vi "Build Get Type.vi"(8 "error in (no error)":errorcluster, 10 "Get Type VI":refnum<vi>, 11 "CS++Actor in":refnum<class "CS++Actor.lvclass">) -> (0 "error out":errorcluster, 3 "CS++Actor out":refnum<class "CS++Actor.lvclass">)   [LabVIEW 2014, in "CS++Actor.lvlib" / "CS++Actor.lvclass"]
uses:
  CS++Actor.lvclass
  CS++Actor.lvclass/CS++Actor.ctl
  <vilib>/Utility/traverseref.llb/TRef TravTarget.ctl
  <vilib>/Utility/traverseref.llb/VI Scripting - Traverse.lvlib
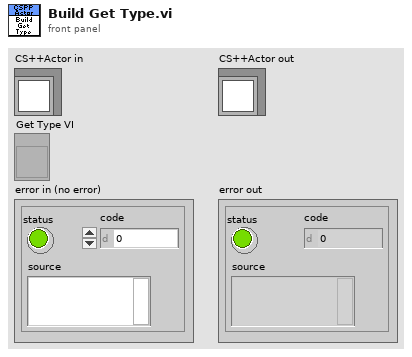
[diagram p1: front panel]
types:
  T1 = enum16{"Replace Class Controls/Indicator", "Connect Unbundler & Bundler"}
  T2 = enum16{"Invalid Wire Rule", "Required", "Recommended", "Optional", "Dynamic Dispatch"}
  T3 = typedef "TRef TravTarget.ctl" = enum16{"FP", "BD", "Other"}
  T4 = typedef "LVRectTypeDef.ctl" = cluster{"Left":i16, "Top":i16, "Right":i16, "Bottom":i16}
  T5 = enum16{"Invalid Wire Rule", "Required", "Recommended", "Optional", "Dynamic Dispatch"}[]
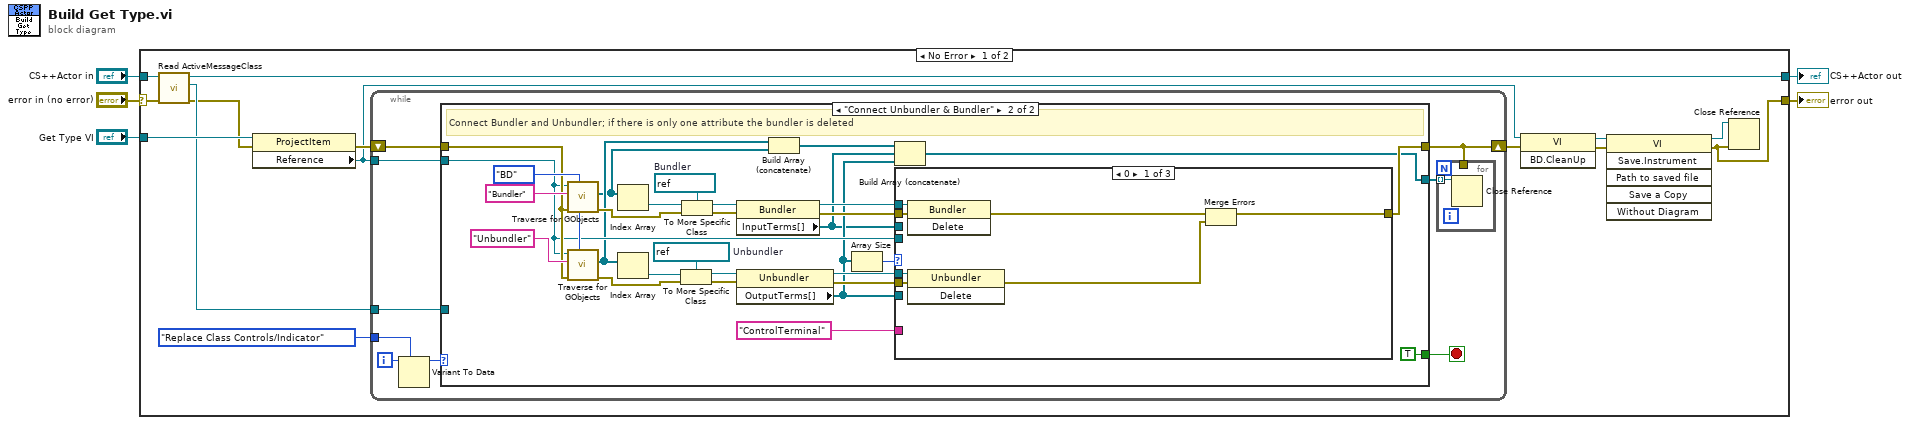
[diagram p0: block diagram]
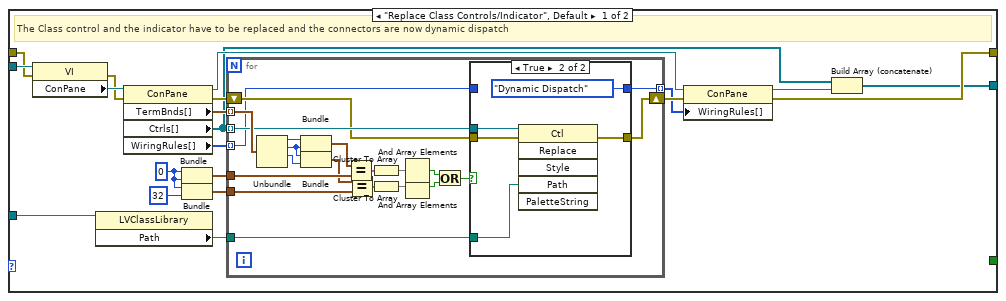
[diagram p2: hidden frame]
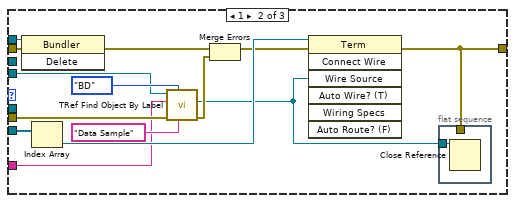
[diagram p4: hidden frame]
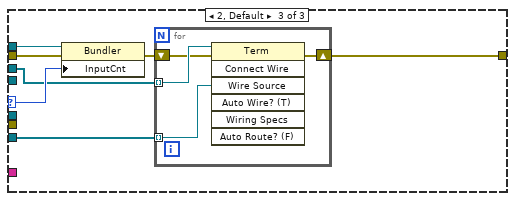
[diagram p5: hidden frame]
diagram:
  n1 = case shown="No Error" "error in (no error)" {
    selector: "error in (no error)" -> [w6 w141]
    tunnel: [w12 w141] -> w4
    tunnel: [w8 w140] -> w2
    tunnel: "CS++Actor in" -> [w7 w140]
    tunnel: "Get Type VI" -> [w18 _]
    frame No Error {
      n2 = call "Read ActiveMessageClass.vi"("error in (no error)"=w6, "CS++Actor in"=w7) -> ("error out"=w9:errorcluster, "ActiveMessageClass"=w10:refnum<vi>, "CS++Actor out"=w8:refnum<class "CS++Actor.lvclass">)  [unwired: 7 in]
      n3 = property class="ProjectItem"(reference=w18, error in=w9) -> (error out=w17:errorcluster, "Reference"=w13:refnum<vi>)  [unwired: 1 out]
      n4 = while {
        tunnel: T1."Replace Class Controls/Indicator" -> [w27]
        tunnel: w13 -> [w24]
        shift-right: [w20] -> w11
        shift-left: w17 -> [w25]
        tunnel: w10 -> [w23]
        i -> [w28]
        stop <- w22 stop-if-true
        n5 = Variant To Data(type=w27, Variant=w28) -> (data=w26:T1)  [unwired: 1 in, 1 out]
        n6 = case shown="\"Connect Unbundler & Bundler\"" w26 {
          tunnel: w25 -> [w48 w96]
          tunnel: w24 -> [w49 w86]
          tunnel: w23 -> [w40 _]
          tunnel: [w35 w85] -> w20
          tunnel: [_ TRUE] -> w22
          tunnel: [w30 w83] -> w21
          frame "Replace Class Controls/Indicator", Default {
            w38 = i16 0
            # "The Class control and the indicator have to be replaced and the connectors are now dynamic dispatch"
            n7 = property class="VI"(reference=w49, error in=w48) -> (error out=w46:errorcluster, "ConPane"=w47:refnum<vi>)  [unwired: 1 out]
            n8 = property class="LVClassLibrary"(reference=w40) -> ("Path"=w39:path)  [unwired: 1 in, 2 out]
            n9 = property class="ConPane"(reference=w47, error in=w46) -> (reference out=w34:refnum<vi>, error out=w44:errorcluster, "TermBnds[]"=w45:T4[], "Ctrls[]"=w32:refnum<vi>[], "WiringRules[]"=w37:T5)
            n10 = Bundle(w38, w38) -> (w42:cluster{i16, i16})  [unwired: 1 in]
            n11 = Bundle(w38, i16 32) -> (w41:cluster{i16, i16})  [unwired: 1 in]
            n12 = for {
              tunnel: w45 -> [w70] mode=indexing
              tunnel: w32 -> [w60] mode=indexing
              shift-right: [w54] -> w36
              shift-left: w44 -> [w59]
              tunnel: w42 -> [w67]
              tunnel: w41 -> [w65]
              tunnel: w39 -> [w55]
              tunnel: w37 -> [w51] mode=indexing
              tunnel: [w50] -> w33 mode=indexing
              n13 = Unbundle(w70) -> ("Left"=w69:i16, "Top"=w52:i16, "Right"=w53:i16)  [unwired: 1 out]
              n14 = Bundle("Left"=w69, "Top"=w52) -> (w68:cluster{"Left":i16, "Top":i16})  [unwired: 1 in]
              n15 = Bundle("Top"=w52, "Right"=w53) -> (w66:cluster{"Top":i16, "Right":i16})  [unwired: 1 in]
              n16 = Equal?(x=w68, y=w67) -> (x = y?=w64:cluster{bool, bool})
              n17 = Equal?(x=w66, y=w65) -> (x = y?=w63:cluster{bool, bool})
              n18 = Cluster To Array(cluster=w64) -> (array=w62:bool[])
              n19 = Cluster To Array(cluster=w63) -> (array=w61:bool[])
              n20 = And Array Elements(Boolean array=w62) -> (logical AND=w58:bool)
              n21 = And Array Elements(Boolean array=w61) -> (logical AND=w57:bool)
              n22 = Or(x=w58, y=w57) -> (x .or. y?=w56:bool)
              n23 = case shown="True" w56 {
                tunnel: w60 -> [_ w77]
                tunnel: w59 -> [w72 w76]
                tunnel: [w72 w75] -> w54
                tunnel: w55 -> [_ w74]
                tunnel: w51 -> [w71 _]
                tunnel: [w71 T2."Dynamic Dispatch" ("Wire Rule")] -> w50
                frame False {
                }
                frame True {
                  n24 = invoke class="Ctl" method="Replace"(reference=w77, error in=w76, "Path"=w74) -> (error out=w75:errorcluster)  [unwired: 3 in, 5 out]
                }
              }
            }
            n25 = property class="ConPane"(reference=w34, error in=w36, "WiringRules[]"=w33) -> (reference out=w31:refnum<vi>, error out=w35:errorcluster)
            n26 = Build Array (concatenate)(w32, w31) -> (w30:refnum<vi>[])
          }
          frame "Connect Unbundler & Bundler" {
            w97 = TRef_TravTarget."BD" ("Traverse Target")
            w102 = refnum<vi> refnum  # Unbundler
            w105 = refnum<vi> refnum  # Bundler
            # "Connect Bundler and Unbundler; if there is only one attribute the bundler is deleted"
            n27 = call <vilib>:"Traverse for GObjects.vi"("Traverse Target"=w97, "error in (no error)"=w96, "Class Name"="Bundler", "VI Refnum"=w86) -> ("error out"=w95:errorcluster, "References"=w81:refnum<vi>[])  [unwired: 4 in, 2 out]
            n28 = call <vilib>:"Traverse for GObjects.vi"("Traverse Target"=w97, "error in (no error)"=w96, "Class Name"="Unbundler", "VI Refnum"=w86) -> ("error out"=w93:errorcluster, "References"=w82:refnum<vi>[])  [unwired: 4 in, 2 out]
            n29 = Index Array(array=w81) -> (element=w94:refnum<vi>)  [unwired: 1 in]
            n30 = Index Array(array=w82) -> (element=w92:refnum<vi>)  [unwired: 1 in]
            n31 = To More Specific Class(target class=w102, reference=w92, error in=w93) -> (specific class reference=w101:refnum<vi>, error out=w100:errorcluster)
            n32 = To More Specific Class(target class=w105, reference=w94, error in=w95) -> (specific class reference=w104:refnum<vi>, error out=w103:errorcluster)
            n33 = property class="Bundler"(reference=w104, error in=w103) -> (reference out=w91:refnum<vi>, error out=w90:errorcluster, "InputTerms[]"=w79:refnum<vi>[])
            n34 = property class="Unbundler"(reference=w101, error in=w100) -> (reference out=w87:refnum<vi>, error out=w89:errorcluster, "OutputTerms[]"=w84:refnum<vi>[])
            n35 = Build Array (concatenate)(w82, w81) -> (w80:refnum<vi>[])
            n36 = Array Size(array=w84) -> (size(s)=w88:i32)
            n37 = Build Array (concatenate)(w80, w79, w84) -> (w83:refnum<vi>[])
            n38 = case shown="0" w88 {
              selector: w88 -> [_ _ w131]
              tunnel: w91 -> [w113 w127 w132]
              tunnel: w90 -> [w112 w126 w134]
              tunnel: w89 -> [w110 w125 _]
              tunnel: w87 -> [w111 _ _]
              tunnel: w84 -> [_ w122 w135]
              tunnel: w86 -> [_ w120 _]
              tunnel: [w109 w115 w130] -> w85
              tunnel: w79 -> [_ _ w129]
              tunnel: "ControlTerminal" ("Class Name") -> [_ w114 _]
              frame 0 {
                n39 = invoke class="Bundler" method="Delete"(reference=w113, error in=w112) -> (error out=w108:errorcluster)  [unwired: 1 in, 2 out]
                n40 = invoke class="Unbundler" method="Delete"(reference=w111, error in=w110) -> (error out=w107:errorcluster)  [unwired: 1 in, 2 out]
                n41 = Merge Errors(w108, w107) -> (w109:errorcluster)
              }
              frame 1 {
                n42 = invoke class="Bundler" method="Delete"(reference=w127, error in=w126) -> (error out=w119:errorcluster)  [unwired: 1 in, 2 out]
                n43 = Index Array(array=w122) -> (element=w121:refnum<vi>)  [unwired: 1 in]
                n44 = call <vilib>:"TRef Find Object By Label.vi"("Label"="Data Sample", "Traverse Target"=TRef_TravTarget."BD", "error in (no error)"=w125, "Class Name"=w114, "VI Ref"=w120) -> ("error out"=w118:errorcluster, "Found Obj Ref"=w116:refnum<vi>)  [unwired: 3 in, 2 out]
                n45 = Merge Errors(w119, w118) -> (w117:errorcluster)
                n46 = invoke class="Term" method="Connect Wire"(reference=w121, error in=w117, "Wire Source"=w116) -> (error out=w115:errorcluster)  [unwired: 4 in, 6 out]
                n47 = flat-sequence {
                  tunnel: w116 -> [w128]
                  tunnel: w115 -> [_]
                  frame #0 {
                    n48 = Close Reference(reference=w128) -> ()  [unwired: 1 in, 1 out]
                  }
                }
              }
              frame 2, Default {
                n49 = property class="Bundler"(reference=w132, error in=w134, "InputCnt"=w131) -> (error out=w133:errorcluster)  [unwired: 1 out]
                n50 = for {
                  tunnel: w135 -> [w136] mode=indexing
                  shift-right: [w137] -> w130
                  shift-left: w133 -> [w138]
                  tunnel: w129 -> [w139] mode=indexing
                  n51 = invoke class="Term" method="Connect Wire"(reference=w139, error in=w138, "Wire Source"=w136) -> (error out=w137:errorcluster)  [unwired: 4 in, 6 out]
                }
              }
            }
          }
        }
        n52 = for {
          tunnel: w21 -> [w29] mode=indexing
          tunnel: w20 -> [_]
          n53 = Close Reference(reference=w29) -> ()  [unwired: 1 in, 1 out]
        }
      }
      n54 = invoke class="VI" method="BD.CleanUp"(reference=w13, error in=w11) -> (reference out=w16:refnum<vi>, error out=w14:errorcluster)  [unwired: 1 in, 1 out]
      n55 = invoke class="VI" method="Save.Instrument"(reference=w16, error in=w14) -> (reference out=w15:refnum<vi>, error out=w12:errorcluster)  [unwired: 4 in, 4 out]
      n56 = Close Reference(reference=w15, error in (no error)=w12) -> ()  [unwired: 1 out]
    }
    frame Error {
    }
  }
  "error out" <- w4
  "CS++Actor out" <- w2
